vi "Address Dialog.vi"(6 "Title":string, 8 "Error In":errorcluster, 11 "Address In":string="localhost") -> (0 "Error Out":errorcluster, 3 "Address Out":string)   [LabVIEW 2018, in "Tests.lvlib"]
uses:
  Tests.lvlib
  <vilib>/Utility/miscctls.llb/LVSelectionTypeDef.ctl
panel:
  out "Host":string="ADDRESS FOR INTEGRATION TESTS"
  in  "Cancel":bool
  in  "OK":bool
  in  "Address":string="localhost"
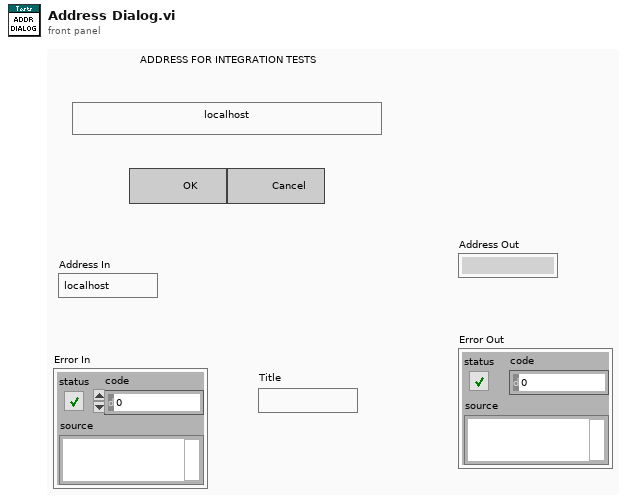
[diagram p1: front panel]
types:
  T1 = typedef "LVSelectionTypeDef.ctl" = cluster{"Selection Start":u32, "Selection End":u32}
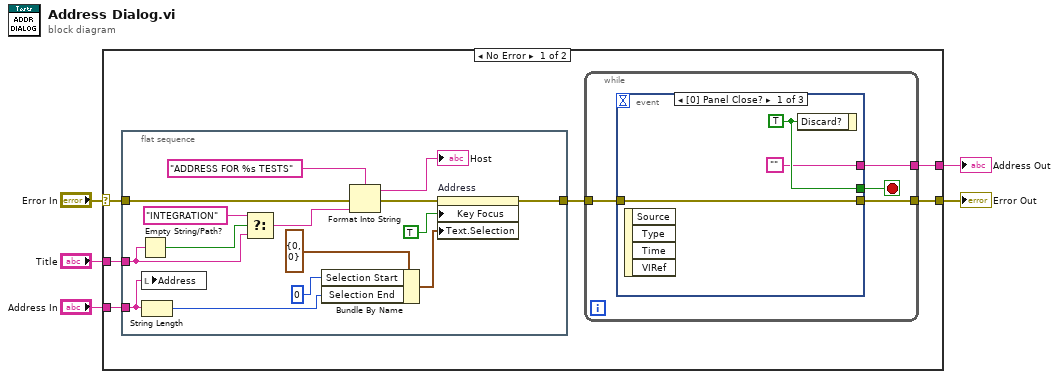
[diagram p0: block diagram]
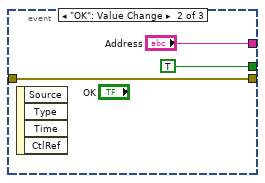
[diagram p2: hidden frame]
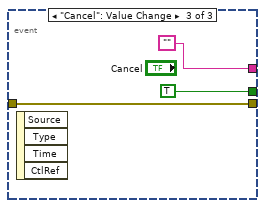
[diagram p3: hidden frame]
diagram:
  n1 = case shown="No Error" "Error In" {
    selector: "Error In" -> [w9 w40]
    tunnel: [w11 w40] -> w4
    tunnel: [w7 _] -> w3
    tunnel: "Address In" -> [w10 _]
    tunnel: "Title" -> [w6 _]
    frame No Error {
      n2 = flat-sequence {
        tunnel: w10 -> [w20]
        tunnel: w9 -> [w26]
        tunnel: [w25] -> w8
        tunnel: w6 -> [w12]
        frame #0 {
          n3 = Empty String/Path?(string/path=w12) -> (empty?=w15:bool)
          n4 = local write "Address"(w20) -> ()
          n5 = String Length(string=w20) -> (length=w19:i32)
          n6 = Select(t="INTEGRATION", s=w15, f=w12) -> (s? t:f=w13:string)
          n7 = Bundle By Name(cluster=T1 {"Selection Start"=0, "Selection End"=0} ("Text.Selection"), "Selection Start"=u32 0, "Selection End"=w19) -> (w22:T1)
          n8 = Format Into String(format string="ADDRESS FOR %s TESTS", error in=w26, w13) -> (resulting string=→"Host":string, error out=w18:errorcluster)  [unwired: 1 in]
          n9 = property on="Address" class="Str"(error in=w18, "Key Focus"=TRUE, "Text.Selection"=w22) -> (error out=w25:errorcluster)  [unwired: 1 in, 1 out]
        }
      }
      n10 = while {
        tunnel: w8 -> [w29]
        tunnel: [w28] -> w11
        tunnel: [w27] -> w7
        stop <- w30 stop-if-true
        n11 = event shown="[0] Panel Close?" {
          selector: _ -> [_ _ _]
          dyn-events: _ -> [_ _ _]
          timeout: _ -> [_ _ _]
          tunnel: [w33 TRUE TRUE] -> w30
          tunnel: w29 -> [w32 w36 w39]
          tunnel: [w32 w36 w39] -> w28
          tunnel: ["" "Address" ""] -> w27
          event Panel Close? {
            w33 = TRUE
            n12 = event-data() -> ()  [unwired: 1 in, 4 out]
            n13 = event-data("Discard?"=w33) -> ()  [unwired: 1 in, 1 out]
          }
          event "OK": Value Change {
            n14 = event-data() -> ()  [unwired: 1 in, 4 out]
          }
          event "Cancel": Value Change {
            n15 = event-data() -> ()  [unwired: 1 in, 4 out]
          }
        }
      }
    }
    frame Error {
    }
  }
  "Error Out" <- w4
  "Address Out" <- w3
